vi "Data 2 Variant.vi"(8 "Error In":errorcluster, 10 "Type Descriptor":string, 11 "Data":i8[](array[numeric])) -> (0 "Error Out":errorcluster, 3 "data":variant)   [LabVIEW 2014, in "CS++DIM.lvlib" / "DIMConnection.lvclass"]
doc: "Convert DIM byte array to variant."
uses:
  DIMConnection.lvclass
  CSPP_Core/Libraries/Utilities/CS++Utilities.lvlib
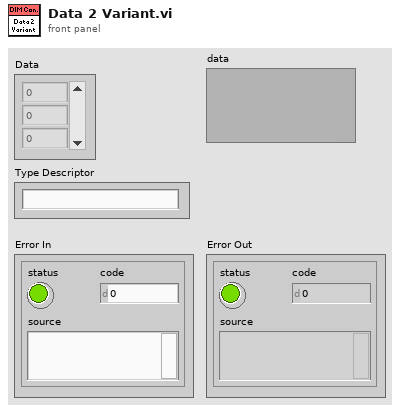
[diagram p1: front panel]
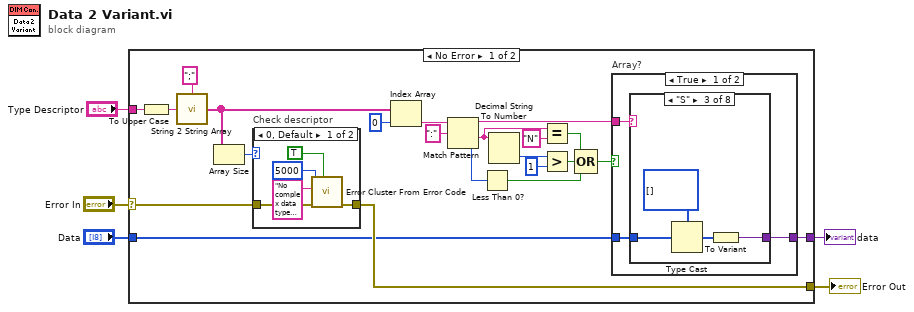
[diagram p0: block diagram]
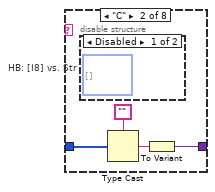
[diagram p3: hidden frame]
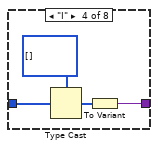
[diagram p5: hidden frame]
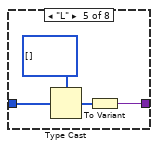
[diagram p6: hidden frame]
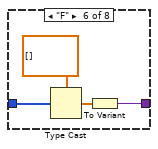
[diagram p7: hidden frame]
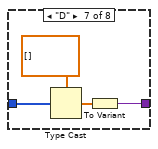
[diagram p8: hidden frame]
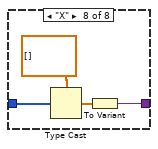
[diagram p9: hidden frame]
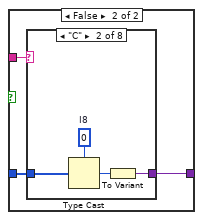
[diagram p10: hidden frame]
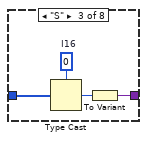
[diagram p12: hidden frame]
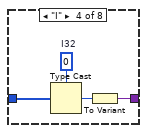
[diagram p13: hidden frame]
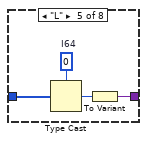
[diagram p14: hidden frame]
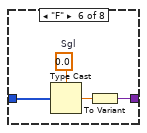
[diagram p15: hidden frame]
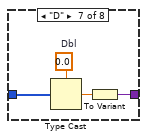
[diagram p16: hidden frame]
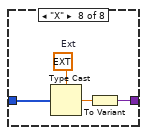
[diagram p17: hidden frame]
diagram:
  n1 = case shown="No Error" "Error In" {
    selector: "Error In" -> [w9 w97]
    tunnel: "Type Descriptor" -> [w25 _]
    tunnel: [w12 w97] -> w4
    tunnel: "Data" -> [w11 w96]
    tunnel: [w10 w96] -> w2
    frame No Error {
      n2 = To Upper Case(1:w25) -> (0:w26:string)
      n3 = call "String 2 String Array.vi"("String"=w26, "Delimiter (\",\")"=";" ("Delimiter (\",\")")) -> ("Substrings"=w23:string[])
      n4 = Array Size(array=w23) -> (size(s)=w24:i32)
      n5 = case "Check descriptor" shown="0, Default" w24 {
        tunnel: w9 -> [w94 w95]
        tunnel: [w93 w95] -> w12
        frame 0, Default {
          n6 = call <vilib>:"Error Cluster From Error Code.vi"("show call chain? (False)"=TRUE, "error in (no error)"=w94, "error message (\"\")"="No complex data types support for now." ("error message (\"\")"), "error code (0)"=5000) -> ("error out"=w93:errorcluster)  [unwired: 5 in]
        }
        frame 1 {
        }
      }
      n7 = Index Array(array=w23, index=0) -> (element=w15:string)
      n8 = Match Pattern(string=w15, regular expression=":") -> (before substring=w13:string, after substring=w8:string, offset past match=w20:i32)  [unwired: 1 in, 1 out]
      n9 = Less Than 0?(x=w20) -> (x < 0?=w16:bool)
      n10 = Decimal String To Number(string=w8) -> (number=w19:i32)  [unwired: 2 in, 1 out]
      n11 = Equal?(x=w8, y="N") -> (x = y?=w6:bool)
      n12 = Greater?(x=w19, y=1) -> (0:w17:bool)
      n13 = Compound Arithmetic op=OR(w6, w17, w16) -> (w14:bool)
      n14 = case "Array?" shown="True" w14 {
        tunnel: w13 -> [w30 w61]
        tunnel: w11 -> [w29 w60]
        tunnel: [w28 w59] -> w10
        frame True {
          n15 = case shown="\"S\"" w30 {
            tunnel: w29 -> [_ w34 w38 w42 w46 w50 w54 w58]
            tunnel: [_ w32 w35 w39 w43 w47 w51 w55] -> w28
            frame Default {
            }
            frame "C" {
              n16 = disable-structure "HB: [I8] vs. Str" shown="Disabled" {
                frame Disabled {
                  (unwired) i8[] []
                }
                frame Enabled {
                }
              }
              n17 = Type Cast(type="", x=w34) -> (*(type *) &x=w33:string)
              n18 = To Variant(anything=w33) -> (Variant=w32:variant)
            }
            frame "S" {
              n19 = Type Cast(type=i16[] [], x=w38) -> (*(type *) &x=w36:i16[])
              n20 = To Variant(anything=w36) -> (Variant=w35:variant)
            }
            frame "I" {
              n21 = Type Cast(type=i32[] [], x=w42) -> (*(type *) &x=w40:i32[])
              n22 = To Variant(anything=w40) -> (Variant=w39:variant)
            }
            frame "L" {
              n23 = Type Cast(type=i64[] [], x=w46) -> (*(type *) &x=w44:i64[])
              n24 = To Variant(anything=w44) -> (Variant=w43:variant)
            }
            frame "F" {
              n25 = Type Cast(type=sgl[] [], x=w50) -> (*(type *) &x=w48:sgl[])
              n26 = To Variant(anything=w48) -> (Variant=w47:variant)
            }
            frame "D" {
              n27 = Type Cast(type=dbl[] [], x=w54) -> (*(type *) &x=w52:dbl[])
              n28 = To Variant(anything=w52) -> (Variant=w51:variant)
            }
            frame "X" {
              n29 = Type Cast(type=ext[] [], x=w58) -> (*(type *) &x=w56:ext[])
              n30 = To Variant(anything=w56) -> (Variant=w55:variant)
            }
          }
        }
        frame False {
          n31 = case shown="\"C\"" w61 {
            tunnel: w60 -> [_ w65 w69 w73 w77 w81 w85 w89]
            tunnel: [_ w63 w67 w71 w75 w79 w83 w87] -> w59
            frame Default {
            }
            frame "C" {
              w62 = i8 0  # I8
              n32 = Type Cast(type=w62, x=w65) -> (*(type *) &x=w64:i8)
              n33 = To Variant(anything=w64) -> (Variant=w63:variant)
            }
            frame "S" {
              w66 = i16 0  # I16
              n34 = Type Cast(type=w66, x=w69) -> (*(type *) &x=w68:i16)
              n35 = To Variant(anything=w68) -> (Variant=w67:variant)
            }
            frame "I" {
              w70 = 0  # I32
              n36 = Type Cast(type=w70, x=w73) -> (*(type *) &x=w72:i32)
              n37 = To Variant(anything=w72) -> (Variant=w71:variant)
            }
            frame "L" {
              w74 = 0  # I64
              n38 = Type Cast(type=w74, x=w77) -> (*(type *) &x=w76:i32)
              n39 = To Variant(anything=w76) -> (Variant=w75:variant)
            }
            frame "F" {
              w78 = sgl 0.0  # Sgl
              n40 = Type Cast(type=w78, x=w81) -> (*(type *) &x=w80:sgl)
              n41 = To Variant(anything=w80) -> (Variant=w79:variant)
            }
            frame "D" {
              w82 = 0.0  # Dbl
              n42 = Type Cast(type=w82, x=w85) -> (*(type *) &x=w84:dbl)
              n43 = To Variant(anything=w84) -> (Variant=w83:variant)
            }
            frame "X" {
              w86 = ext 0.0  # Ext
              n44 = Type Cast(type=w86, x=w89) -> (*(type *) &x=w88:ext)
              n45 = To Variant(anything=w88) -> (Variant=w87:variant)
            }
          }
        }
      }
    }
    frame Error {
    }
  }
  "data" <- w2
  "Error Out" <- w4
